vi "SMS Candidate Selection Example.vi"() -> ()   [LabVIEW 2020]
panel:
  out "ROI":u16[][](graph)
  in  "ROI Index":i32
  in  "Quit":bool
  in  "Blink Sensitivity":sgl=1.3
  out "Candidate Image":T1(plugin-control)
  out "Read Image":T1(plugin-control)
  in  "Image to Read":path=path "C:/Users/User/Documents/MATLAB/Candidate Selection/PAINT Images/Color01_00009.tif"
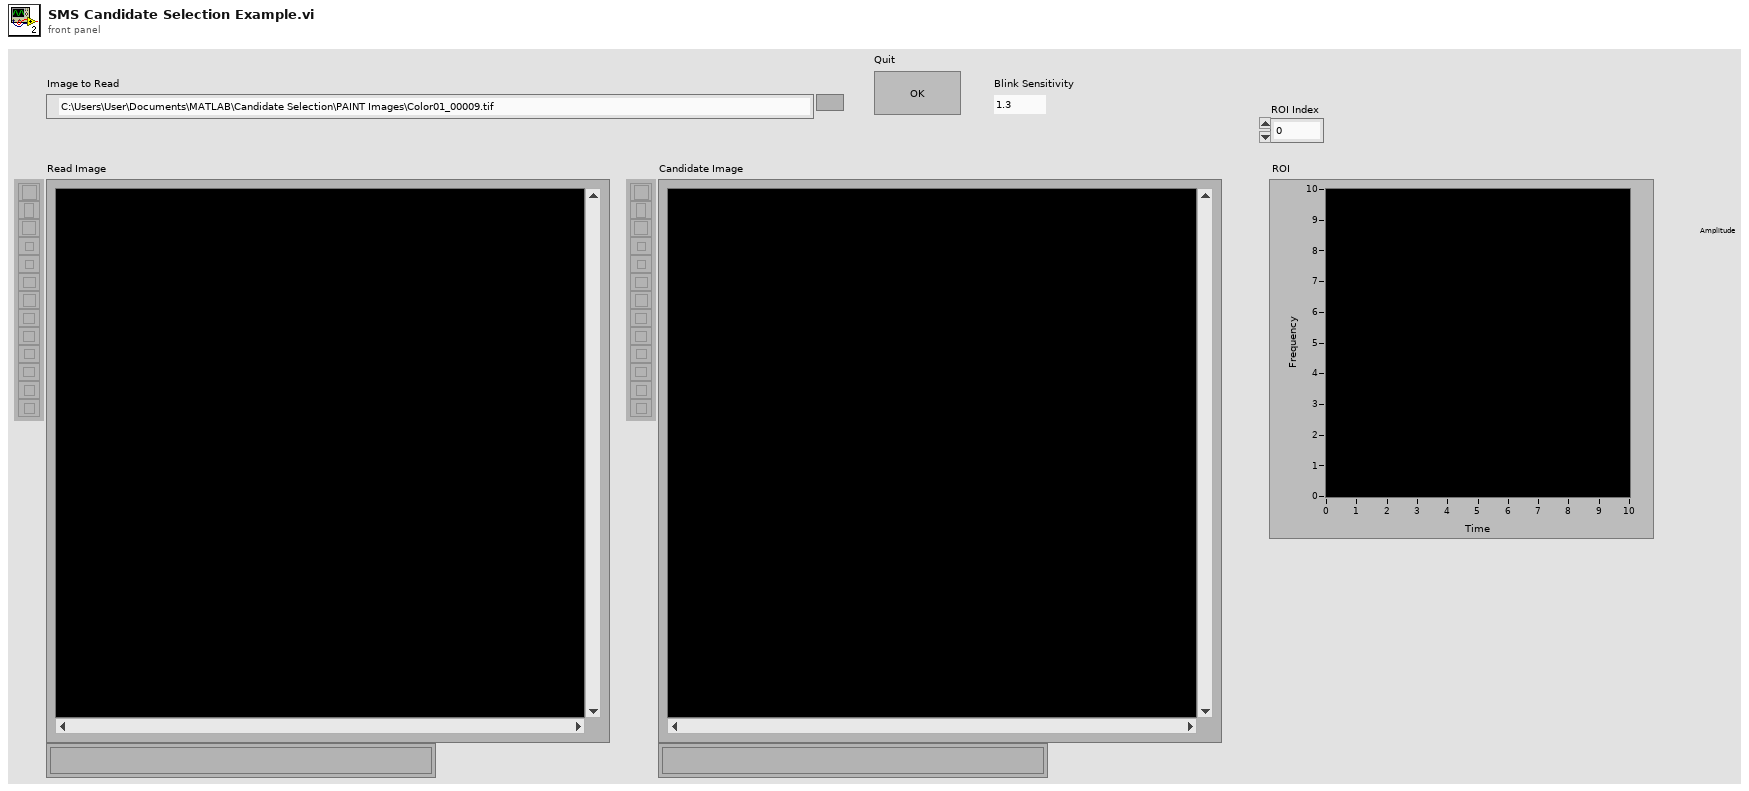
[diagram p1: front panel]
types:
  T1 = typedef "IMAQ Image.ctl" = refnum<image>
  T2 = typedef "Image Type" = u32
  T3 = cluster{"Global Rectangle":i32[], "Contours":cluster{"Contour Type":u32, "ROI Type":u32, "Points":i32[]}[]}
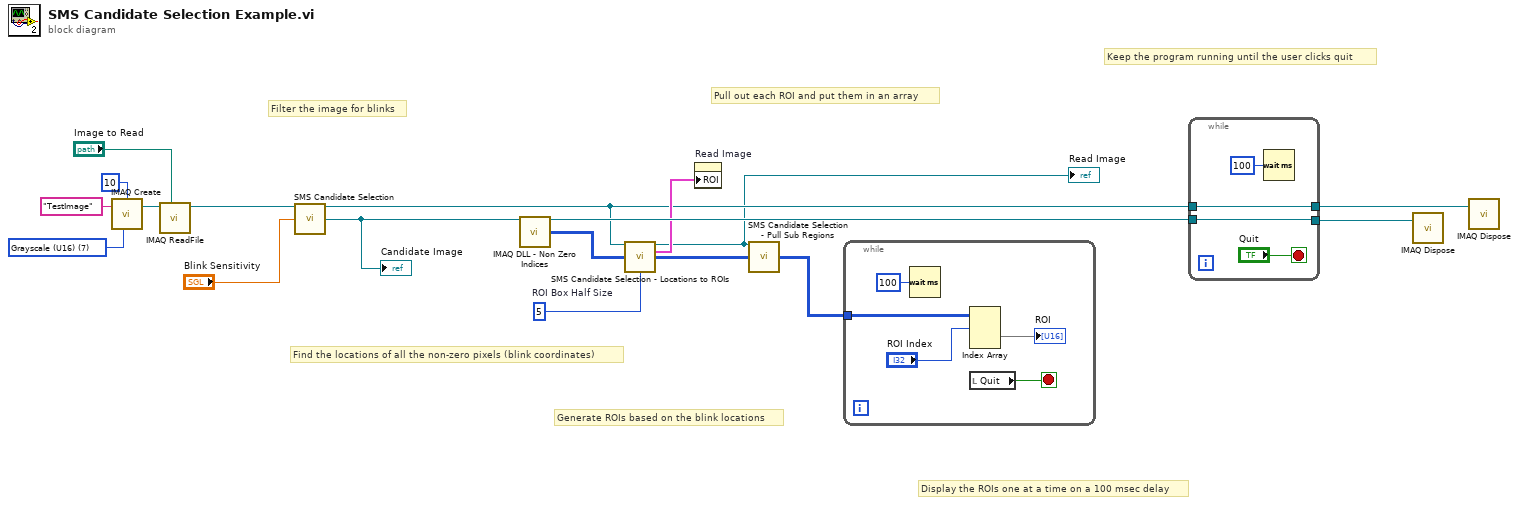
[diagram p0: block diagram]
diagram:
  w6 = u8 5  # ROI Box Half Size
  w17 = T2 7 items=["Grayscale (U8)", "Grayscale (I16)", "Grayscale (SGL)", "Complex (CSG)", "RGB (U32)", "HSL (U32)", "RGB (U64)", "Grayscale (U16)"] ("Image Type")
  # "Keep the program running until the user clicks quit"
  # "Display the ROIs one at a time on a 100 msec delay"
  # "Pull out each ROI and put them in an array"
  # "Generate ROIs based on the blink locations"
  # "Find the locations of all the non-zero pixels (blink coordinates)"
  # "Filter the image for blinks"
  n1 = call "IMAQ Create"("Border Size"=10, "Image Name"="TestImage", "Image Type"=w17) -> ("New Image"=w18:T1)  [unwired: 2 in, 1 out]
  n2 = call "IMAQ ReadFile"("File Path"="Image to Read", "Image"=w18) -> ("Image Out"=w13:T1)  [unwired: 5 in, 4 out]
  n3 = call "SMS Candidate Selection.vi"("Image Ref (U16)"=w13, "Blink Sensitivity"="Blink Sensitivity") -> ("Image Ref (U16) - Dup"=w5:T1, "Cadidate Image Ref"=w9:T1)  [unwired: 11 in, 1 out]
  "Candidate Image" <- w9
  n4 = call "IMAQ DLL - Non Zero Indices.vi"("IMAQ Ref"=w9) -> ("IMAQ Ref (Dup)"=w10:T1, "Row Column Indices"=w8:i32[][])  [unwired: 11 in, 2 out]
  n5 = call "SMS Candidate Selection - Locations to ROIs.vi"("Image Ref"=w5, "Row Column Indices"=w8, "Box Half Size"=w6) -> ("Image Ref (DUP)"=w1:T1, "Image ROIs"=w7:T3, "ROI Coordinates (Left, Top, Right, Bottom)"=w4:i32[][])  [unwired: 9 in, 1 out]
  "Read Image" <- w1
  n6 = property on="Read Image" class="ImageControl"("ROI"=w7) -> ()  [unwired: 2 in, 2 out]
  n7 = call "SMS Candidate Selection - Pull Sub Regions.vi"("Image Ref"=w1, "ROI Coordinates"=w4) -> ("ROIs"=w3:u16[][][])  [unwired: 11 in, 2 out]
  n8 = while {
    tunnel: w3 -> [w22]
    stop <- w23 stop-if-true
    n9 = Wait (ms)(milliseconds to wait=u32 100) -> ()  [unwired: 1 out]
    n10 = Index Array(array=w22, index (dim 0)="ROI Index") -> (element=→"ROI":u16[][])  [unwired: 2 in]
    n11 = local read "Quit"() -> (w23:bool)
  }
  n12 = while {
    tunnel: [w27] -> w11
    tunnel: w10 -> [w27]
    tunnel: w5 -> [w26]
    tunnel: [w26] -> w12
    stop <- "Quit" stop-if-true
    n13 = Wait (ms)(milliseconds to wait=u32 100) -> ()  [unwired: 1 out]
  }
  n14 = call "IMAQ Dispose"("Image"=w11) -> ()  [unwired: 5 in, 1 out]
  n15 = call "IMAQ Dispose"("Image"=w12) -> ()  [unwired: 5 in, 1 out]
